vi "TestCheesyDrive.vi"() -> ()   [LabVIEW 2016]
panel:
  in  "negInertiaScalar":dbl=4.0
  in  "WheelNonLinearity":dbl=0.65
  out "Waveform Chart":cluster{"Left PWM":dbl, "Right PWM":dbl}(graph)
  in  "Throttle":dbl(slide)=0.007874015748031496 scale=-1.0..1.0
  in  "Wheel":dbl(slide) scale=-1.0..1.0
  in  "Quickturn":bool
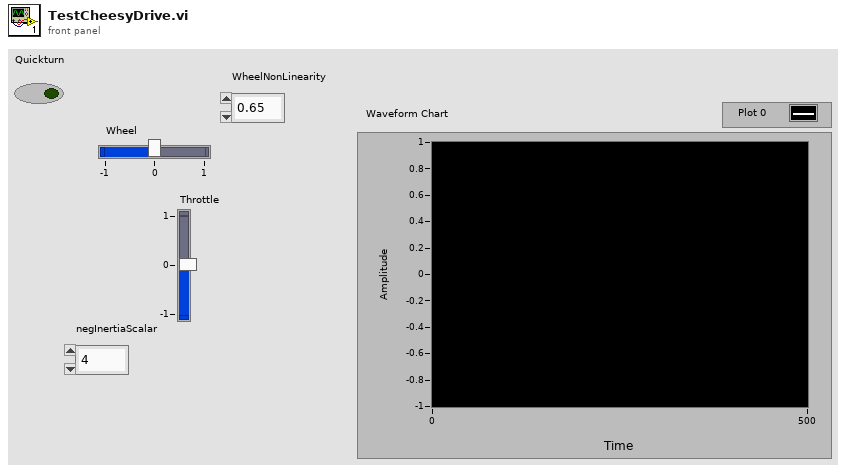
[diagram p1: front panel]
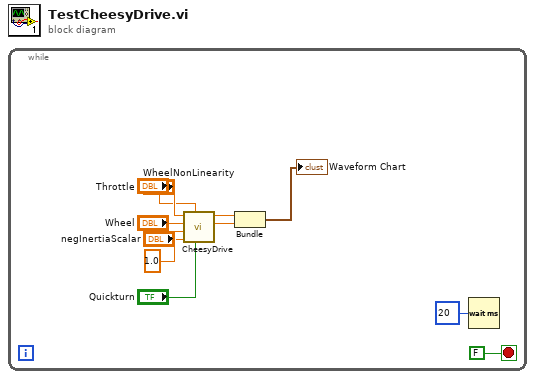
[diagram p0: block diagram]
diagram:
  n1 = while {
    stop <- FALSE stop-if-true
    n2 = call "CheesyDrive.vi"("Quickturn"="Quickturn", "WheelNonLinearity"="WheelNonLinearity", "negInertiaScalar"="negInertiaScalar", "Sensitivty"=1.0, "Wheel"="Wheel", "Throttle"="Throttle") -> ("Right PWM"=w6:dbl, "Left PWM"=w7:dbl)  [unwired: 4 in]
    n3 = Bundle("Left PWM"=w7, "Right PWM"=w6) -> (→"Waveform Chart":cluster{"Left PWM":dbl, "Right PWM":dbl})  [unwired: 1 in]
    n4 = Wait (ms)(milliseconds to wait=u32 20) -> ()  [unwired: 1 out]
  }
